vi "Get LV Class Path by Name.vi"(8 "error in (no error)":errorcluster, 11 "class name":string) -> (0 "error out":errorcluster, 3 "class path":path)   [LabVIEW 2015, in "Scripting.lvlib"]
uses:
  Scripting.lvlib
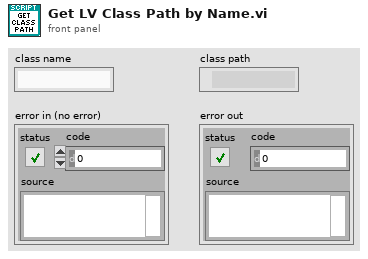
[diagram p1: front panel]
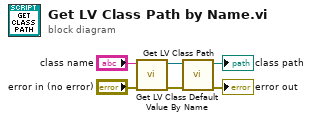
[diagram p0: block diagram]
diagram:
  n1 = call <vilib>:"Get LV Class Default Value By Name.vi"("error in (no error)"="error in (no error)", "class name"="class name") -> ("error out"=w1:errorcluster, "object"=w2:refnum<class>)  [unwired: 8 in]
  n2 = call <vilib>:"Get LV Class Path.vi"("error in (no error)"=w1, "object"=w2) -> ("error out"=→"error out":errorcluster, "class path"=→"class path":path)  [unwired: 8 in]
